vi "_subtract value.vi"(6 "label":T1, 8 "i":errorcluster, 10 "B":refnum<class "Value.lvclass">, 11 "A":refnum<class "Value.lvclass">) -> (0 "error out":errorcluster, 2 "c":refnum<class "Value.lvclass">, 3 "A out":refnum<class "Value.lvclass">)   [LabVIEW 2023, in "LabGRAD.lvlib" / "Value.lvclass"]
uses:
  Value.lvclass
  Value.lvclass/Value.ctl
  operation.ctl
  UiObjects/string control.ctl
  UiObjects/UiObjects.lvclass
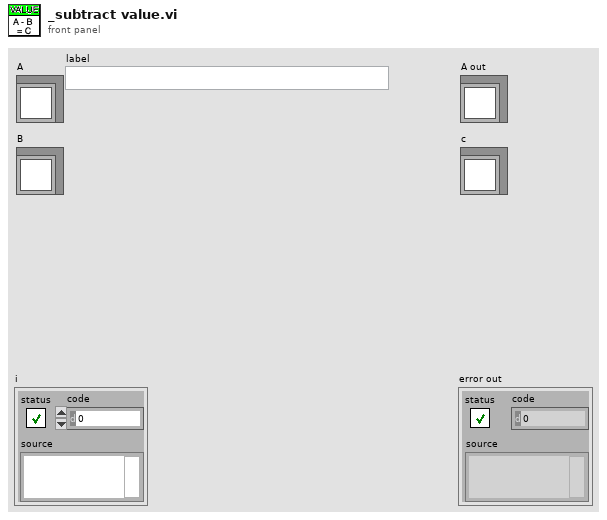
[diagram p1: front panel]
types:
  T1 = typedef "UiObjects.lvlib/UiObjects.lvclass/string control.ctl" = string
  T2 = typedef "LabGRAD.lvlib/Value.lvclass/operation.ctl" = enum16{"nop", "add", "subtract", "power", "multiply", "divide", "tanh"}
  T3 = typedef "UiObjects.lvlib/UiObjects.lvclass/numeric value control.ctl" = dbl
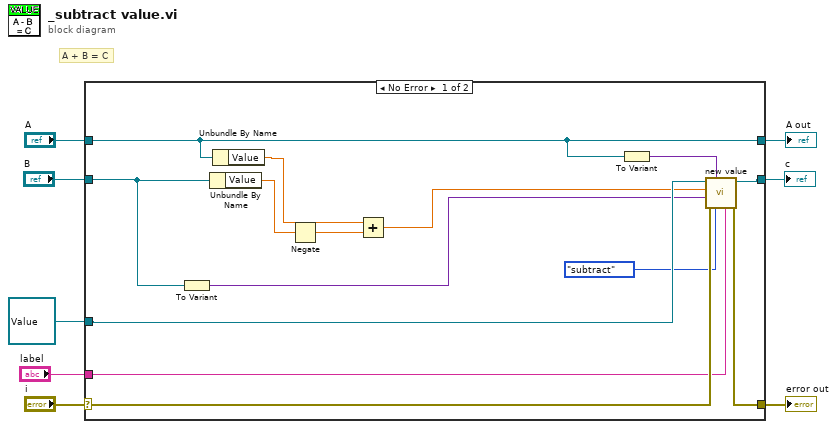
[diagram p0: block diagram]
diagram:
  # "A + B = C"
  n1 = case shown="No Error" "i" {
    selector: "i" -> [w13 w25]
    tunnel: [w12 w25] -> w7
    tunnel: [w16 w24] -> w5
    tunnel: "A" -> [w16 w24]
    tunnel: "B" -> [w20 _]
    tunnel: [w14 w23] -> w3
    tunnel: refnum<class "Value.lvclass"> refnum ("B") -> [w19 w23]
    tunnel: "label" -> [w10 _]
    frame No Error {
      n2 = To Variant(anything=w20) -> (Variant=w17:variant)
      n3 = Unbundle By Name(w20) -> ("Value"=w21:T3)
      n4 = Unbundle By Name(w16) -> ("Value"=w22:T3)
      n5 = Negate(x=w21) -> (-x=w9:T3)
      n6 = Add(x=w22, y=w9) -> (x+y=w18:T3)
      n7 = To Variant(anything=w16) -> (Variant=w15:variant)
      n8 = call "new value.vi"("Label"=w10, "operation"=operation."subtract", "Previous"=w15, "error in (no error)"=w13, "Other"=w17, "data"=w18, "Value in"=w19) -> ("error out"=w12:errorcluster, "Value out"=w14:refnum<class "Value.lvclass">)  [unwired: 3 in]
    }
    frame Error {
    }
  }
  "error out" <- w7
  "A out" <- w5
  "c" <- w3
